vi "Ballard XML Generator.Open Message Buffer.vi"(9 "name":string, 10 "id":string, 11 "string in":string) -> (3 "string out":string)   [LabVIEW 2020]
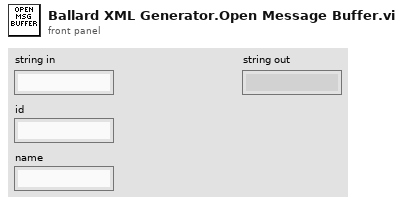
[diagram p1: front panel]
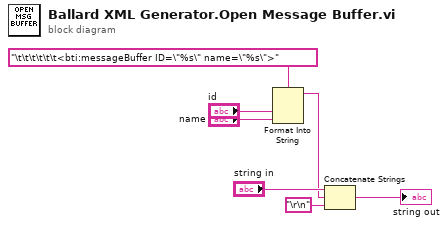
[diagram p0: block diagram]
diagram:
  n1 = Format Into String(format string="\t\t\t\t\t\t<bti:messageBuffer ID=\"%s\" name=\"%s\">", "id", "name") -> (resulting string=w3:string)  [unwired: 2 in, 1 out]
  n2 = Concatenate Strings("string in", w3, "\r\n") -> (→"string out":string)
